vi "Configure Standard Waveform [STD].vi"(4 "dc offset (0.00 V)":dbl[unit] format="%.3f", 5 "start phase (0.00 Degrees)":dbl[unit] format="%.3f", 6 "amplitude (1.00 V)":dbl[unit]=1.0 format="%.3f", 7 "frequency (1000.0 Hz)":dbl[unit]=1000.0 format="%^.2e", 8 "error in (no error)":errorcluster, 9 "waveform (Sine)":i32(ring)=1 items=["Sine"=1, "Square"=2, "Triangle"=3, "Ramp Up"=4, "Ramp Down"=5, "DC"=6], 10 "channel name (\"CHANNEL1\")":string="CHANNEL1", 11 "CS++Fgen in":refnum<class "CS++Fgen.lvclass">) -> (0 "error out":errorcluster, 3 "CS++Fgen out":refnum<class "CS++Fgen.lvclass">)   [LabVIEW 2013, in "CS++Fgen.lvlib" / "CS++Fgen.lvclass"]
doc: "This VI configures the properties of the function generator that affect standard waveform generation. These properties are the waveform, amplitude, DC offset, frequency, and start phase.\n\nNotes:\n\n(1) This VI is part of the IviFgenStdFunc [STD] extension group."
uses:
  CS++Fgen.lvclass
  Core/Classes/CS++ProcessVariables/ProcessVariable/PV.lvclass
  CS++Fgen.lvclass/CS++Fgen.ctl
  Core/Classes/CS++ProcessVariables/PVConnection/PVConnection.lvclass
  Core/Classes/CS++ProcessVariables/ProcessVariable/PV.lvclass/PV.ctl
  Core/Classes/CS++ProcessVariables/ProcessVariable/Write Data.vi
  Core/Classes/CS++ProcessVariables/ProcessVariable/Write Timestamp.vi
  Core/Classes/CS++ProcessVariables/ProcessVariable/Write Quality.vi
  Core/Classes/CS++ProcessVariables/ProcessVariable/Write status.vi
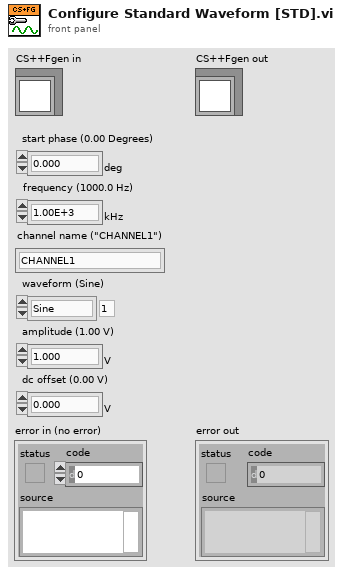
[diagram p1: front panel]
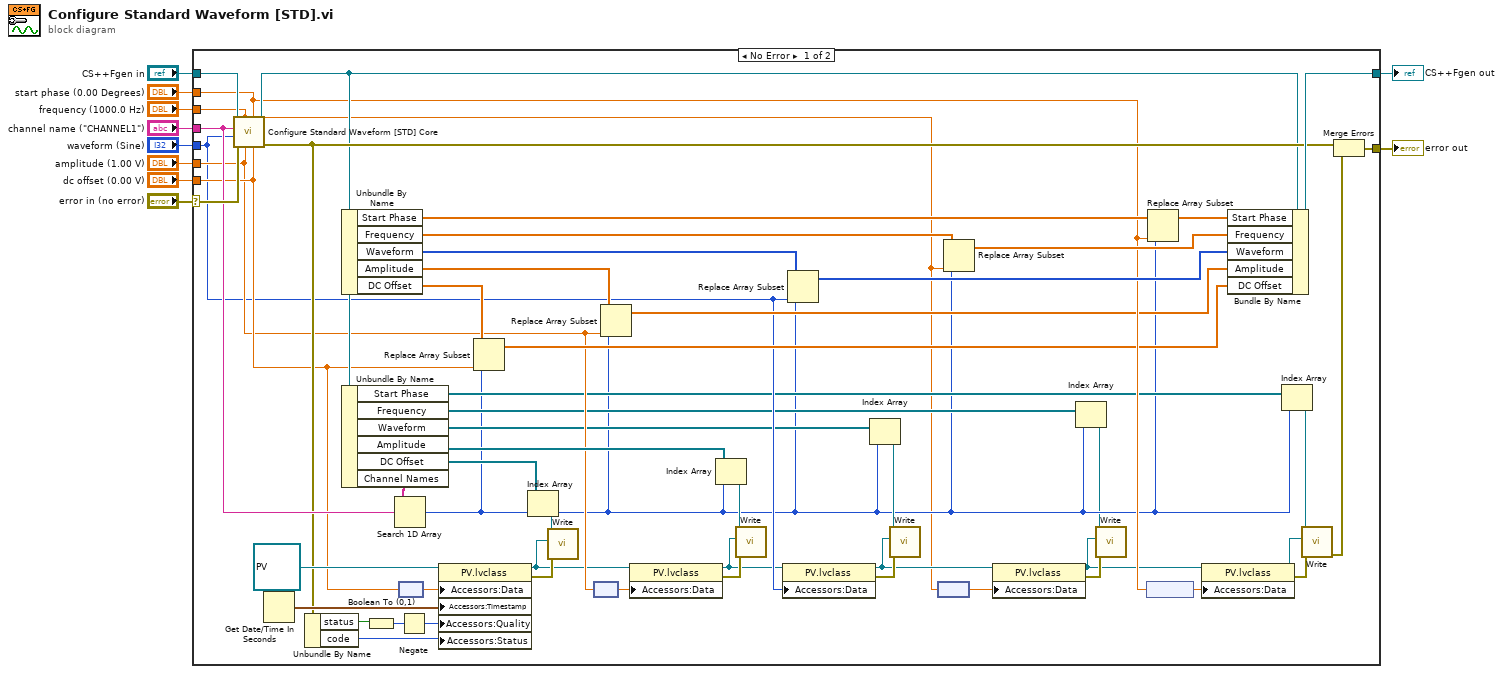
[diagram p0: block diagram]
diagram:
  n1 = case shown="No Error" "error in (no error)" {
    selector: "error in (no error)" -> [w64 w67]
    tunnel: [w45 w67] -> w9
    tunnel: [w47 w66] -> w7
    tunnel: "CS++Fgen in" -> [w65 w66]
    tunnel: "channel name (\"CHANNEL1\")" -> [w48 _]
    tunnel: "start phase (0.00 Degrees)" -> [w38 _]
    tunnel: "frequency (1000.0 Hz)" -> [w11 _]
    tunnel: "dc offset (0.00 V)" -> [w32 _]
    tunnel: "waveform (Sine)" -> [w24 _]
    tunnel: "amplitude (1.00 V)" -> [w27 _]
    frame No Error {
      n2 = call-dynamic "Configure Standard Waveform [STD] Core.vi"("dc offset (0.00 V)"=w32, "start phase (0.00 Degrees)"=w38, "amplitude (1.00 V)"=w27, "frequency (1000.0 Hz)"=w11, "error in (no error)"=w64, "waveform (Sine)"=w24, "channel name (\"CHANNEL1\")"=w48, "CS++Fgen in"=w65) -> ("error out"=w46:errorcluster, "CS++Fgen out"=w44:refnum<class "CS++Fgen.lvclass">)  [unwired: 2 in]
      n3 = Get Date/Time In Seconds() -> (seconds since 1Jan1904=w63:timestamp)
      n4 = Unbundle By Name(w46) -> ("status"=w57:bool, "code"=w55:i32)
      n5 = Unbundle By Name(w44) -> ("Start Phase"=w40:dbl[unit][], "Frequency"=w43:dbl[unit][], "Waveform"=w42:i32[], "Amplitude"=w36:dbl[unit][], "DC Offset"=w35:dbl[unit][])
      n6 = Unbundle By Name(w44) -> ("Start Phase"=w20:refnum<class "PVConnection.lvclass">[], "Frequency"=w18:refnum<class "PVConnection.lvclass">[], "Waveform"=w22:refnum<class "PVConnection.lvclass">[], "Amplitude"=w50:refnum<class "PVConnection.lvclass">[], "DC Offset"=w59:refnum<class "PVConnection.lvclass">[], "Channel Names"=w60:string[])
      n7 = Boolean To (0,1)(Boolean=w57) -> (0, 1=w56:i16)
      n8 = Search 1D Array(1D array=w60, element=w48) -> (index of element=w17:i32)  [unwired: 1 in]
      n9 = node(w32) -> (w31:dbl)
      n10 = Negate(x=w56) -> (-x=w54:i16)
      n11 = property class="PV.lvclass"(reference=refnum<class "PV.lvclass"> refnum ("PV"), "Accessors:Data"=w31, "Accessors:Timestamp"=w63, "Accessors:Quality"=w54, "Accessors:Status"=w55) -> (reference out=w26:refnum<class "PV.lvclass">, error out=w61:errorcluster)  [unwired: 1 in]
      n12 = Replace Array Subset(array=w35, new element=w32, index=w17) -> (w33:dbl[unit][])
      n13 = Index Array(array=w59, index=w17) -> (element=w58:refnum<class "PVConnection.lvclass">)
      n14 = call-dynamic "Write.vi"("error in (no error)"=w61, "PV"=w26, "PVConnection in"=w58) -> ()  [unwired: 7 in, 2 out]
      n15 = node(w27) -> (w30:dbl)
      n16 = Replace Array Subset(array=w36, new element=w27, index=w17) -> (w34:dbl[unit][])
      n17 = property class="PV.lvclass"(reference=w26, "Accessors:Data"=w30) -> (reference out=w23:refnum<class "PV.lvclass">, error out=w29:errorcluster)  [unwired: 1 in]
      n18 = Index Array(array=w50, index=w17) -> (element=w28:refnum<class "PVConnection.lvclass">)
      n19 = call-dynamic "Write.vi"("error in (no error)"=w29, "PV"=w23, "PVConnection in"=w28) -> ()  [unwired: 7 in, 2 out]
      n20 = property class="PV.lvclass"(reference=w23, "Accessors:Data"=w24) -> (reference out=w13:refnum<class "PV.lvclass">, error out=w25:errorcluster)  [unwired: 1 in]
      n21 = Replace Array Subset(array=w42, new element=w24, index=w17) -> (w53:i32[])
      n22 = Index Array(array=w22, index=w17) -> (element=w21:refnum<class "PVConnection.lvclass">)
      n23 = call-dynamic "Write.vi"("error in (no error)"=w25, "PV"=w13, "PVConnection in"=w21) -> ()  [unwired: 7 in, 2 out]
      n24 = node(w11) -> (w16:dbl)
      n25 = Replace Array Subset(array=w43, new element=w11, index=w17) -> (w41:dbl[unit][])
      n26 = property class="PV.lvclass"(reference=w13, "Accessors:Data"=w16) -> (reference out=w12:refnum<class "PV.lvclass">, error out=w15:errorcluster)  [unwired: 1 in]
      n27 = Index Array(array=w18, index=w17) -> (element=w14:refnum<class "PVConnection.lvclass">)
      n28 = call-dynamic "Write.vi"("error in (no error)"=w15, "PV"=w12, "PVConnection in"=w14) -> ()  [unwired: 7 in, 2 out]
      n29 = node(w38) -> (w37:dbl)
      n30 = Replace Array Subset(array=w40, new element=w38, index=w17) -> (w39:dbl[unit][])
      n31 = property class="PV.lvclass"(reference=w12, "Accessors:Data"=w37) -> (reference out=w52:refnum<class "PV.lvclass">, error out=w51:errorcluster)  [unwired: 1 in]
      n32 = Bundle By Name(cluster=w44, "Start Phase"=w39, "Frequency"=w41, "Waveform"=w53, "Amplitude"=w34, "DC Offset"=w33) -> (w47:refnum<class "CS++Fgen.lvclass">)
      n33 = Index Array(array=w20, index=w17) -> (element=w19:refnum<class "PVConnection.lvclass">)
      n34 = call-dynamic "Write.vi"("error in (no error)"=w51, "PV"=w52, "PVConnection in"=w19) -> ("error out"=w49:errorcluster)  [unwired: 7 in, 1 out]
      n35 = Merge Errors(w46, w49) -> (w45:errorcluster)
    }
    frame Error {
    }
  }
  "error out" <- w9
  "CS++Fgen out" <- w7
